vi "WLAN Configure Common.vi"(0 "Instrument Handle In":refnum<k21>, 1 "Selector String":string, 5 "Common Configuration":T1={"Center Frequency (Hz)"=1000000000.0, "Reference Level (dBm)"=0.0, "External Attenuation (dB)"=0.0, "Trigger Enabled"=TRUE, "Digital Trigger Source"="PXI_Trig0", "Trigger Delay (s)"=0.0, "Selected Ports"=""} {"Trigger Delay (s)" format="%.2p"; "External Attenuation (dB)" format="%.2f"; "Reference Level (dBm)" format="%.2f"; "Center Frequency (Hz)" format="%.6p"}, 11 "error in (no error)":errorcluster) -> (4 "Instrument Handle Out":refnum<k21>, 15 "error out":errorcluster)   [LabVIEW 2016, in "RFmxWLAN.lvlib"]
uses:
  RFmxWLAN.lvlib
  Common/SA Common Configuration.ctl
  <vilib>/RFmx/WLAN/mx/RFmxWLAN.llb/RFmxWLAN Configure Digital Edge Trigger.vi
  <resource>/objmgr/RFmxWLAN.rc
  Common/Common.lvlib
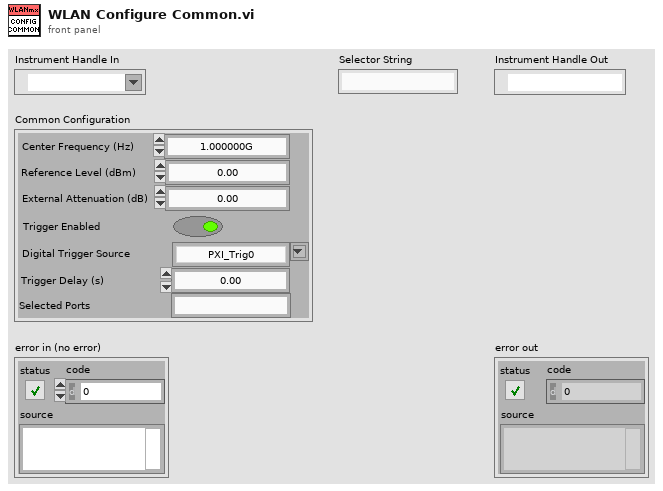
[diagram p1: front panel]
types:
  T1 = typedef "Common.lvlib/SA Common Configuration.ctl" = cluster{"Center Frequency (Hz)":dbl, "Reference Level (dBm)":dbl, "External Attenuation (dB)":dbl, "Trigger Enabled":bool, "Digital Trigger Source":string, "Trigger Delay (s)":dbl, "Selected Ports":string}
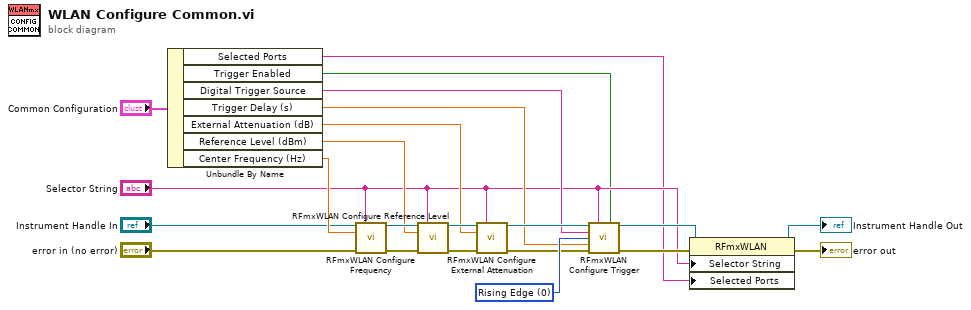
[diagram p0: block diagram]
diagram:
  w17 = 0 items=["Rising Edge", "Falling Edge"] ("Digital Edge")
  n1 = Unbundle By Name("Common Configuration") -> ("Selected Ports"=w1:string, "Trigger Enabled"=w2:bool, "Digital Trigger Source"=w8:string, "Trigger Delay (s)"=w7:dbl, "External Attenuation (dB)"=w18:dbl, "Reference Level (dBm)"=w14:dbl, "Center Frequency (Hz)"=w19:dbl)
  n2 = call <vilib>:"RFmxWLAN Configure Frequency.vi"("Instrument Handle In"="Instrument Handle In", "Selector String"="Selector String", "Center Frequency (Hz)"=w19, "error in (no error)"="error in (no error)") -> ("Instrument Handle Out"=w16:refnum<k21>, "error out"=w15:errorcluster)  [unwired: 10 in]
  n3 = call <vilib>:"RFmxWLAN Configure Reference Level.vi"("Instrument Handle In"=w16, "Selector String"="Selector String", "Reference Level"=w14, "error in (no error)"=w15) -> ("Instrument Handle Out"=w20:refnum<k21>, "error out"=w21:errorcluster)  [unwired: 10 in]
  n4 = call <vilib>:"RFmxWLAN Configure External Attenuation.vi"("Instrument Handle In"=w20, "Selector String"="Selector String", "External Attenuation (dB)"=w18, "error in (no error)"=w21) -> ("Instrument Handle Out"=w13:refnum<k21>, "error out"=w12:errorcluster)  [unwired: 10 in]
  n5 = call-poly <vilib>:"RFmxWLAN Configure Trigger.vi"("Instrument Handle In"=w13, "Selector String"="Selector String", "Enable Trigger?"=w2, "Digital Edge Source"=w8, "Digital Edge"=w17, "Trigger Delay (s)"=w7, "error in (no error)"=w12) -> ("Instrument Handle Out"=w5:refnum<k21>, "error out"=w11:errorcluster)  [unwired: 7 in]
  n6 = property class="RFmxWLAN"(reference=w5, error in=w11, "Selector String"="Selector String", "Selected Ports"=w1) -> (reference out=→"Instrument Handle Out":refnum<k21>, error out=→"error out":errorcluster)
